vi "Read Measured Table Reference.vi"(8 "error in (no error)":errorcluster, 11 "AnalogInput in":refnum<class "AnalogInput.lvclass">) -> (0 "error out":errorcluster, 2 "Measured Table Reference":refnum<vi>, 3 "AnalogInput out":refnum<class "AnalogInput.lvclass">)   [LabVIEW 2019, in "AnalogInput.lvlib" / "AnalogInput.lvclass"]
uses:
  Library/AnalogInput.lvclass
  Library/AnalogInput.lvclass/AnalogInput.ctl
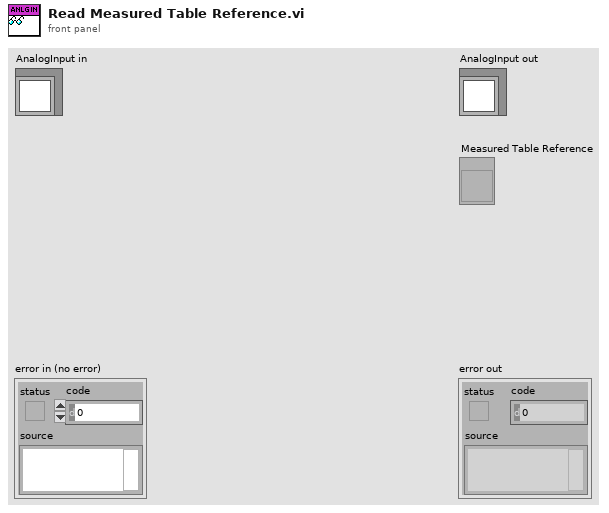
[diagram p1: front panel]
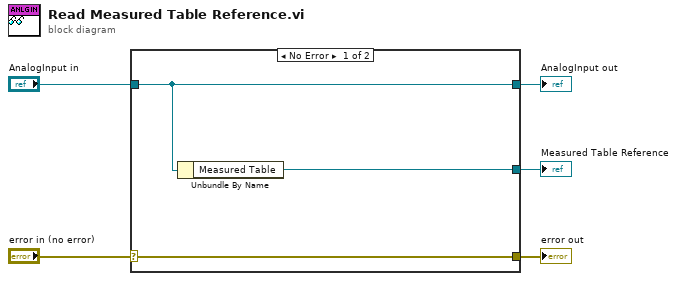
[diagram p0: block diagram]
diagram:
  n1 = case shown="No Error" "error in (no error)" {
    selector: "error in (no error)" -> [w8 w9]
    tunnel: [w8 w9] -> w4
    tunnel: [w7 w10] -> w2
    tunnel: "AnalogInput in" -> [w7 w10]
    tunnel: [w6 _] -> w1
    frame No Error {
      n2 = Unbundle By Name(w7) -> ("Measured Table"=w6:refnum<vi>)
    }
    frame Error {
    }
  }
  "error out" <- w4
  "AnalogInput out" <- w2
  "Measured Table Reference" <- w1
